vi "Read CCDF (Trace).vi"(8 "error in (no error)":errorcluster, 11 "VISA resource name":refnum<visa-resource-name>) -> (0 "error out":errorcluster, 1 "Peak Power Value":dbl, 2 "Average Power Value":dbl, 3 "VISA resource name out":refnum<visa-resource-name>, 5 "Peak-to-average Power Value":dbl)   [LabVIEW 2014, in "Agilent U2000 Series.lvlib"]
doc: "Retrieves the power value of the CCDF trace.\n\nNote:\nThis VI is not applicable for U2040 X-Series."
uses:
  Agilent U2000 Series.lvlib
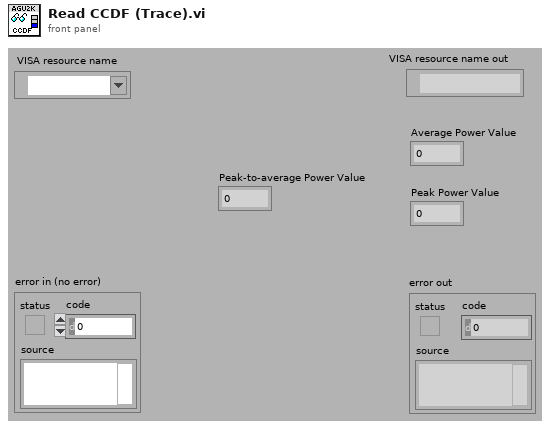
[diagram p1: front panel]
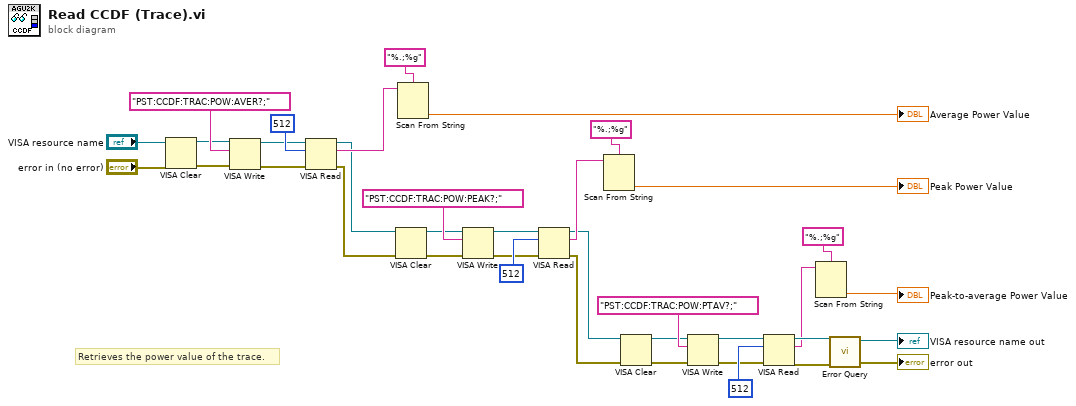
[diagram p0: block diagram]
diagram:
  # "Retrieves the power value of the trace."
  n1 = VISA Clear(VISA resource name="VISA resource name", error in (no error)="error in (no error)") -> (VISA resource name out=w36:refnum<visa-resource-name>, error out=w35:errorcluster)
  n2 = VISA Write(VISA resource name=w36, write buffer="PST:CCDF:TRAC:POW:AVER?;", error in (no error)=w35) -> (VISA resource name out=w9:refnum<visa-resource-name>, error out=w27:errorcluster)  [unwired: 1 out]
  n3 = VISA Read(VISA resource name=w9, byte count=u32 512, error in (no error)=w27) -> (VISA resource name out=w8:refnum<visa-resource-name>, read buffer=w32:string, error out=w10:errorcluster)  [unwired: 1 out]
  n4 = VISA Clear(VISA resource name=w8, error in (no error)=w10) -> (VISA resource name out=w29:refnum<visa-resource-name>, error out=w28:errorcluster)
  n5 = Scan From String(format string="%.;%g", input string=w32) -> (output 1=→"Average Power Value":dbl)  [unwired: 2 in, 4 out]
  n6 = VISA Write(VISA resource name=w29, write buffer="PST:CCDF:TRAC:POW:PEAK?;", error in (no error)=w28) -> (VISA resource name out=w25:refnum<visa-resource-name>, error out=w24:errorcluster)  [unwired: 1 out]
  n7 = VISA Read(VISA resource name=w25, byte count=u32 512, error in (no error)=w24) -> (VISA resource name out=w13:refnum<visa-resource-name>, read buffer=w22:string, error out=w12:errorcluster)  [unwired: 1 out]
  n8 = Scan From String(format string="%.;%g", input string=w22) -> (output 1=→"Peak Power Value":dbl)  [unwired: 2 in, 4 out]
  n9 = VISA Clear(VISA resource name=w13, error in (no error)=w12) -> (VISA resource name out=w19:refnum<visa-resource-name>, error out=w18:errorcluster)
  n10 = VISA Write(VISA resource name=w19, write buffer="PST:CCDF:TRAC:POW:PTAV?;", error in (no error)=w18) -> (VISA resource name out=w16:refnum<visa-resource-name>, error out=w15:errorcluster)  [unwired: 1 out]
  n11 = VISA Read(VISA resource name=w16, byte count=u32 512, error in (no error)=w15) -> (VISA resource name out=w5:refnum<visa-resource-name>, read buffer=w1:string, error out=w2:errorcluster)  [unwired: 1 out]
  n12 = Scan From String(format string="%.;%g", input string=w1) -> (output 1=→"Peak-to-average Power Value":dbl)  [unwired: 2 in, 4 out]
  n13 = call "Error Query.vi"("error in (no error)"=w2, "VISA resource name"=w5) -> ("error out"=→"error out":errorcluster, "VISA resource name out"=→"VISA resource name out":refnum<visa-resource-name>)  [unwired: 8 out]
